vi "List Title.vi"(8 "error in (no error)":errorcluster, 11 "List Processes View Model in":refnum<class "List Processes View Model.lvclass">) -> (0 "error out":errorcluster, 2 "Title":string, 3 "List Processes View Model out":refnum<class "List Processes View Model.lvclass">)   [LabVIEW 2020, in "List Processes View Model.lvclass"]
uses:
  List Processes View Model.lvclass
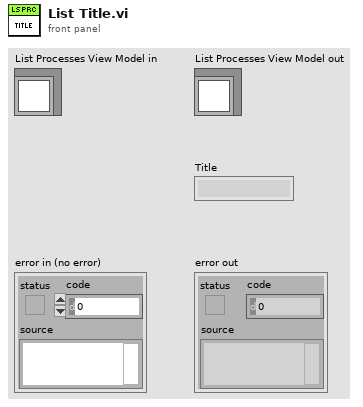
[diagram p1: front panel]
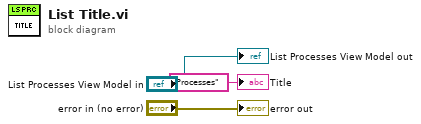
[diagram p0: block diagram]
diagram:
  "error out" <- "error in (no error)"
  "List Processes View Model out" <- "List Processes View Model in"
  "Title" <- "Processes" ("Title")
